vi "tester.vi"() -> ()   [LabVIEW 2016]
uses:
  JSON RPC.lvclass
panel:
  in  "error in (no error)":errorcluster
  out "error out":errorcluster
  out "JSON string":string
  in  "params":string[](array[string])
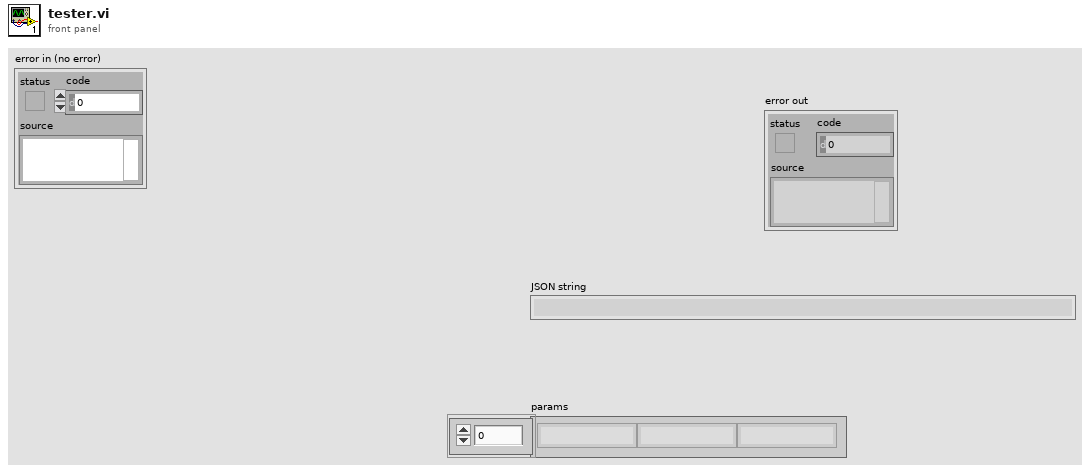
[diagram p1: front panel]
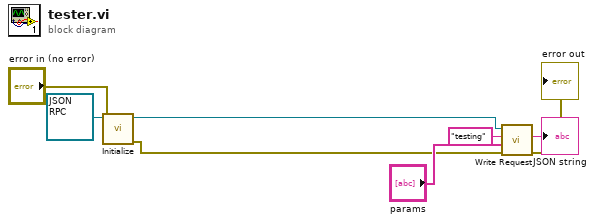
[diagram p0: block diagram]
diagram:
  n1 = call-dynamic "Initialize.vi"("error in (no error)"="error in (no error)", "JSON RPC in"=refnum<class "JSON RPC.lvclass"> refnum) -> ("error out"=w3:errorcluster, "JSON RPC out"=w7:refnum<class "JSON RPC.lvclass">)  [unwired: 8 in]
  n2 = call-dynamic "Write Request.vi"("error in (no error)"=w3, "params"="params", "method"="testing", "JSON RPC in"=w7) -> ("error out"=→"error out":errorcluster, "JSON string"=→"JSON string":string)  [unwired: 5 in, 1 out]
